vi "Configure Level.vi"(0 "VISA resource name":refnum<visa-resource-name>, 1 "Reference Level (dBm)":dbl, 2 "Reference Level Offset (dB)":dbl, 5 "Amplitude Units":u16(ring) items=["dBm", "dBmV", "dBmA", "dBuV", "dBuVm", "dBuA", "dBuAm", "dBpt", "dBg", "Volts", "Watts", "Amps"], 7 "Input Impedance":u16(ring) items=["50", "75"], 11 "error in (no error)":errorcluster, 12 "Enable Auto Attenuation":bool=TRUE, 13 "Manual Attenuation (dB)":dbl=30.0, 14 "Attenuation Step (B)":i32=2) -> (4 "VISA resource name out":refnum<visa-resource-name>, 15 "error out":errorcluster)   [LabVIEW 2014]
uses:
  Agilent ESA PSA Series.lvlib
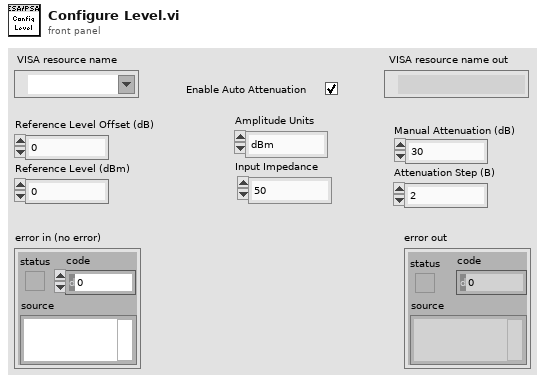
[diagram p1: front panel]
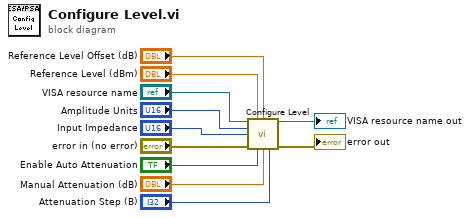
[diagram p0: block diagram]
diagram:
  n1 = call "Configure Level.vi"("VISA resource name"="VISA resource name", "Reference Level (0)"="Reference Level (dBm)", "Reference Level Offset (0 dB)"="Reference Level Offset (dB)", "Amplitude Units (0: dBm)"="Amplitude Units", "Input Impedance (0: 50 ohms)"="Input Impedance", "error in (no error)"="error in (no error)", "Enable Auto Attenuation (T: Enable)"="Enable Auto Attenuation", "Manual Attenuation (30 dB)"="Manual Attenuation (dB)", "Attenuation Step (2 dB)"="Attenuation Step (B)") -> ("VISA resource name out"=→"VISA resource name out":refnum<visa-resource-name>, "error out"=→"error out":errorcluster)  [unwired: 5 in]
